vi "Parse {} UnescapedVariable-Text.vi"(8 "Error In":errorcluster) -> (0 "Error Out":errorcluster)   [LabVIEW 2018, in "Tests.lvlib" / "Parser.lvlib"]
uses:
  Parser.lvlib
  src/Toolkit/Tokens/Text/Text.lvclass
  src/Toolkit/Tokens/UnescapedVariable/UnescapedVariable.lvclass
  src/Toolkit/Tokens/Keyable/API/Keyable.lvclass/Keyable.ctl
  src/Toolkit/Tokens/Keyable/API/Read Key.vi
  src/Toolkit/Readers/String/String.lvclass
  D:/Users/cfield/Code/Field R&D Services/Mustache/trunk/src/Toolkit/Readers/Abstract/Abstract.lvclass
  <vilib>/Utility/LVClass/Get LV Class Name.vi
  src/Toolkit/Tokens/Text/API/Read Content.vi
  <vilib>/addons/_JKI Toolkits/Caraya/classes/Assert/Assert Equal_Variant.vi
  src/Toolkit/Tokens/Keyable/API/Keyable.lvclass
  <vilib>/addons/_JKI Toolkits/Caraya/classes/Test/Test.lvclass
  src/Toolkit/Parser/Parser.lvclass
  <vilib>/addons/_JKI Toolkits/Caraya/classes/Assert/Assert.lvclass
  src/Toolkit/Tokens/Abstract/Abstract.lvclass
  Tests.lvlib
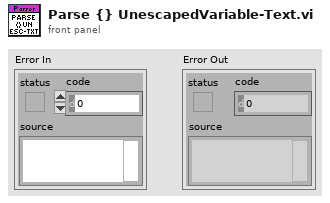
[diagram p1: front panel]
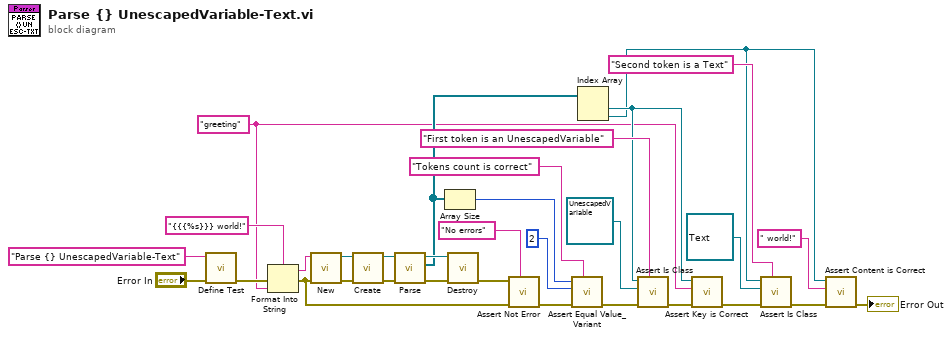
[diagram p0: block diagram]
diagram:
  w3 = "greeting" ("String")
  n1 = call <vilib>:"Define Test.vi"("error in (no error)"="Error In", "Label (VI Title)"="Parse {} UnescapedVariable-Text") -> ("error out"=w23:errorcluster)  [unwired: 9 in]
  n2 = Format Into String(format string="{{{%s}}} world!", error in=w23, w3) -> (resulting string=w13:string, error out=w15:errorcluster)  [unwired: 1 in]
  n3 = call "New.vi"("Error In"=w15, "String"=w13) -> ("Error Out"=w29:errorcluster, "String"=w30:refnum<class "String.lvclass">)  [unwired: 8 in]
  n4 = call "Create.vi"("Error In"=w29, "Reader"=w30) -> ("Error Out"=w28:errorcluster, "Parser"=w27:refnum<class "Parser.lvclass">)  [unwired: 8 in]
  n5 = call "Parse.vi"("Error In"=w28, "Parser In"=w27) -> ("Error Out"=w25:errorcluster, "Tokens"=w16:refnum<class "Abstract.lvclass">[], "Parser Out"=w26:refnum<class "Parser.lvclass">)  [unwired: 7 in]
  n6 = Array Size(array=w16) -> (size(s)=w19:i32)
  n7 = call "Destroy.vi"("Error In"=w25, "Parser"=w26) -> ("Error Out"=w24:errorcluster)  [unwired: 8 in, 1 out]
  n8 = call <vilib>:"Assert Not Error.vi"("Label"="No errors", "error in (no error)"=w15, "Not Error?"=w24) -> ("error out"=w21:errorcluster)  [unwired: 8 in]
  n9 = call <vilib>:"Assert Equal Value_Variant.vi"("Label"="Tokens count is correct", "error in (no error)"=w21, "Y"=2 ("size(s)"), "X"=w19) -> ("error out"=w17:errorcluster)  [unwired: 7 in]
  n10 = Index Array(array=w16) -> (element #1=w5:refnum<class "Abstract.lvclass">, element #2=w1:refnum<class "Abstract.lvclass">)  [unwired: 2 in]
  n11 = call "Assert Is Class.vi"("Label"="First token is an UnescapedVariable", "Error In"=w17, "Expected"=refnum<class "UnescapedVariable.lvclass"> refnum ("Mustache.lvlib:Tokens.lvlib:UnescapedVariable.lvclass"), "Actual"=w5) -> ("Error Out"=w4:errorcluster)  [unwired: 7 in]
  n12 = call "Assert Key is Correct.vi"("Error In"=w4, "Expected"=w3, "Token"=w5) -> ("Error Out"=w12:errorcluster)  [unwired: 8 in]
  n13 = call "Assert Is Class.vi"("Label"="Second token is a Text", "Error In"=w12, "Expected"=refnum<class "Text.lvclass"> refnum ("Mustache.lvlib:Tokens.lvlib:Text.lvclass"), "Actual"=w1) -> ("Error Out"=w11:errorcluster)  [unwired: 7 in]
  n14 = call "Assert Content is Correct.vi"("Error In"=w11, "Expected"=" world!", "Token"=w1) -> ("Error Out"=→"Error Out":errorcluster)  [unwired: 8 in]
